vi "array_to_string.vi"(7 "delimiter (Tab)":string, 10 "Array of Strings":string[](array[string])) -> (1 "delimited string":string)   [LabVIEW 2024]
doc: "Converts 1D Array of strings to a delimited string"
uses:
  <userlib>/_OpenG.lib/string/string.llb/openg_string.lvlib
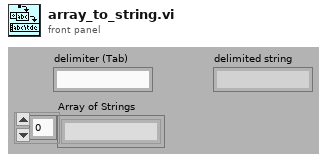
[diagram p1: front panel]
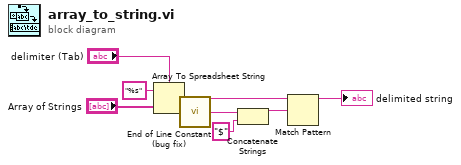
[diagram p0: block diagram]
diagram:
  n1 = Array To Spreadsheet String(delimiter (Tab)="delimiter (Tab)", array="Array of Strings", 3:"%s" ("format string")) -> (spreadsheet string=w2:string)
  n2 = call <userlib>:"End of Line Constant (bug fix).vi"() -> ("Platform EOL"=w1:string)  [unwired: 5 in]
  n3 = Concatenate Strings(w1, "$" ("Substring")) -> (w3:string)
  n4 = Match Pattern(string=w2, regular expression=w3) -> (before substring=→"delimited string":string)  [unwired: 1 in, 3 out]
